vi "FRCts20_Backend_FGVDates.vi"(10 "Date":timestamp, 11 "Command":T1=enum."Get Day") -> (1 "FirstDate":string, 2 "Dates":timestamp[](array[timestamp]), 3 "Day":i32)   [LabVIEW 2013, in "FRCts20_Backend_Engine_Deprecated.lvlib"]
uses:
  FRCts20_Backend_Engine_Deprecated.lvlib
  FRCts20_Backend_FGVDatesCommands.ctl
  FRCts20_Backend_Controls.lvlib
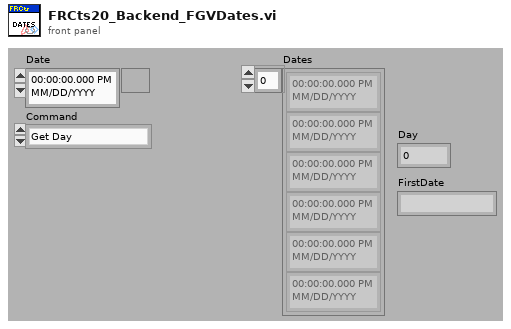
[diagram p1: front panel]
types:
  T1 = typedef "FRCts20_Backend_Controls.lvlib/FRCts20_Backend_FGVDatesCommands.ctl" = enum16{"Set Dates", "Get Day", "Get First Day"}
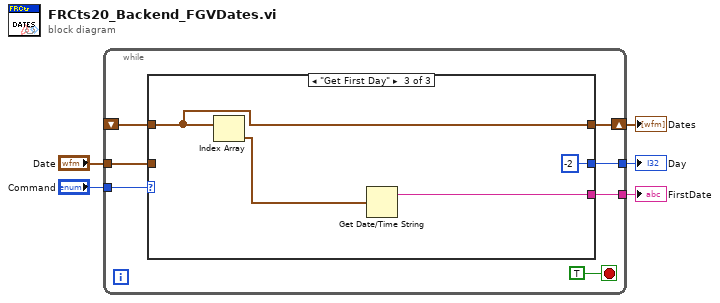
[diagram p0: block diagram]
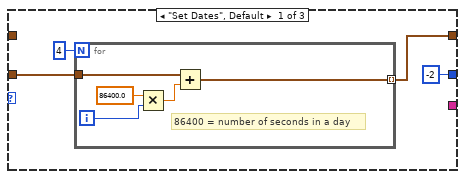
[diagram p2: hidden frame]
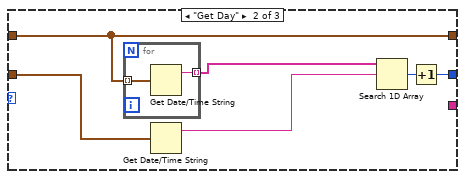
[diagram p3: hidden frame]
diagram:
  n1 = while {
    tunnel: "Command" -> [w11]
    tunnel: "Date" -> [w10]
    shift-right: [w8] -> w2
    shift-left: _ -> [w9]
    tunnel: [w7] -> w3
    tunnel: [w6] -> w1
    stop <- TRUE stop-if-true
    n2 = case shown="\"Get First Day\"" w11 {
      tunnel: w10 -> [w16 w24 _]
      tunnel: w9 -> [_ w25 w32]
      tunnel: [w14 w25 w32] -> w8
      tunnel: [-2 ("index of element") w26 -2 ("index of element")] -> w7
      tunnel: [_ _ w30] -> w6
      frame "Set Dates", Default {
        n3 = for {
          N: 4 -> [_]
          tunnel: w16 -> [w21]
          tunnel: [w17] -> w14 mode=indexing
          i -> [w19]
          # "86400 = number of seconds in a day"
          n4 = Multiply(x=86400.0, y=w19) -> (x*y=w18:dbl)
          n5 = Add(x=w21, y=w18) -> (x+y=w17:timestamp)
        }
      }
      frame "Get Day" {
        n6 = for {
          tunnel: w25 -> [w29] mode=indexing
          tunnel: [w28] -> w23 mode=indexing
          n7 = Get Date/Time String(seconds (now)=w29) -> (date string=w28:string)  [unwired: 2 in, 1 out]
        }
        n8 = Get Date/Time String(seconds (now)=w24) -> (date string=w22:string)  [unwired: 2 in, 1 out]
        n9 = Search 1D Array(1D array=w23, element=w22) -> (index of element=w27:i32)  [unwired: 1 in]
        n10 = Increment(x=w27) -> (x+1=w26:i32)
      }
      frame "Get First Day" {
        n11 = Index Array(array=w32) -> (element=w33:timestamp)  [unwired: 1 in]
        n12 = Get Date/Time String(seconds (now)=w33) -> (date string=w30:string)  [unwired: 2 in, 1 out]
      }
    }
  }
  "Day" <- w3
  "Dates" <- w2
  "FirstDate" <- w1
